vi "Actor Core.vi"(8 "error in":errorcluster, 11 "Off-Grid in":refnum<class "Off-Grid.lvclass">) -> (0 "error out":errorcluster, 3 "Actor out":refnum<class "Actor.lvclass">)   [LabVIEW 2018, in "Off-Grid Actor.lvlib" / "Off-Grid.lvclass"]
doc: "(<B>Filename</B>: Actor Framework.lvlib:Actor.lvclass:Actor Core.vi)\n\nReceives messages to the actor, reacts to them, and initiates any error handling that may shut the actor down.\n\nDescendant classes may override this VI to append parallel tasks for the actor to complete while it handles messages. Overrides use the Call Parent Method node."
uses:
  Off-Grid.lvclass
  C:/Users/Administrator/Desktop/LabVIEW EMS/Optimization/Generic Optimization Actor/Generic Optimization/Generic Optimization.lvclass
  C:/Program Files (x86)/National Instruments/LabVIEW 2018/vi.lib/ActorFramework/Actor/Actor.lvclass
  C:/Users/Administrator/Desktop/LabVIEW EMS/EMS Generic Actor/EMS Generic/EMS Generic.lvclass
  <vilib>/ActorFramework/Actor/Actor.lvclass
  Generic Optimization Actor/Generic Optimization Messages/Find and Rejoin Devices Msg/Find and Rejoin Devices Msg.lvclass
  C:/Program Files (x86)/National Instruments/LabVIEW 2018/vi.lib/ActorFramework/Message/Message.lvclass
  <vilib>/ActorFramework/Actor/Actor.lvclass/Actor.ctl
  <vilib>/ActorFramework/Message Enqueuer/Message Enqueuer.lvclass/Message Enqueuer.ctl
  EMS Generic Actor/EMS Generic/EMS Generic.lvclass/EMS Generic.ctl
  Generic Optimization Actor/Generic Optimization/Optimization Controls/PCC Data.ctl
  <vilib>/ActorFramework/Message Enqueuer/Init from Existing Queue.vi
  <vilib>/ActorFramework/Message Enqueuer/Message Enqueuer.lvclass
  Generic Optimization Actor/Generic Optimization/Generic Optimization.lvclass
  EMS Generic Actor/EMS Generic/EMS Generic.lvclass
panel:
  out "Solution Result":string="Waiting"
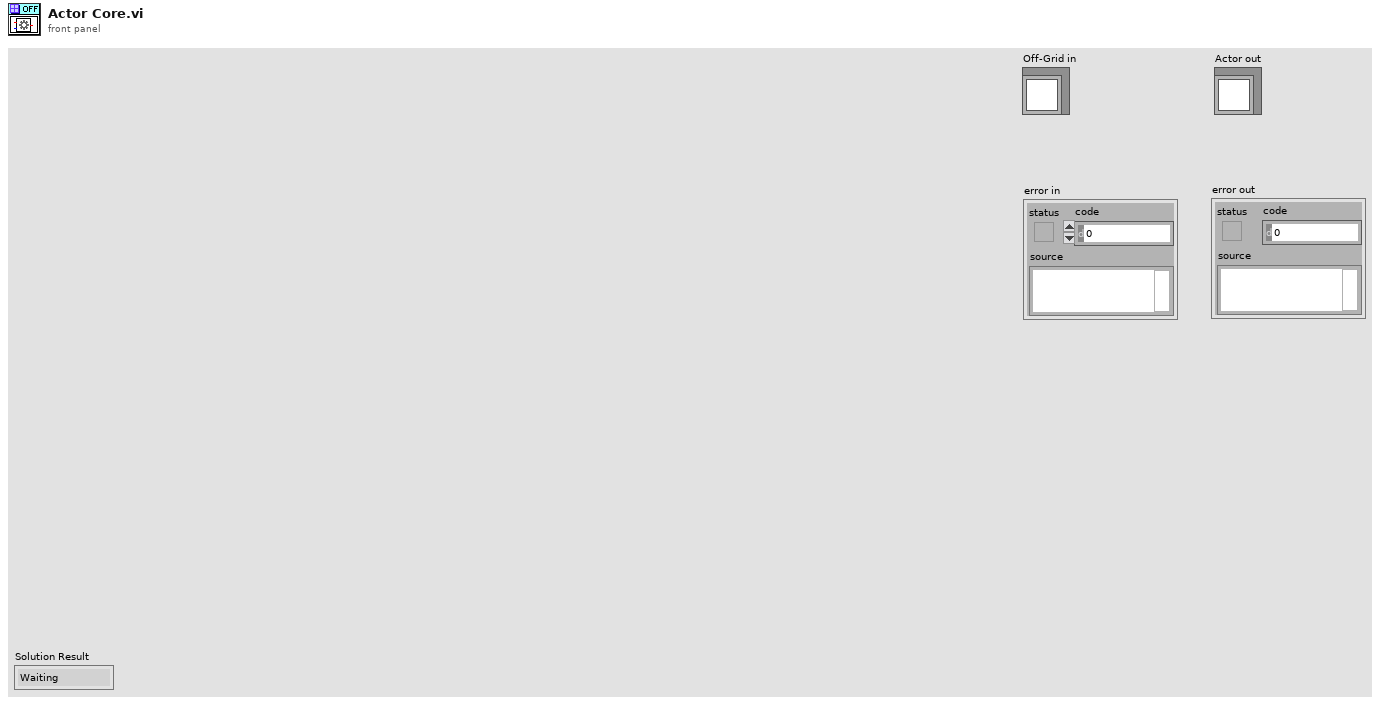
[diagram p1: front panel]
types:
  T1 = typedef "CSEISMIC DDS.lvlib/CSEISMIC DDS.lvclass/DeviceID.ctl" = string
  T2 = typedef "Generic Optimization Actor.lvlib/Generic Optimization.lvclass/Bus by ID.ctl" = cluster{"DeviceID":T1, "Bus ID":dbl}
  T3 = typedef "Generic Optimization Actor.lvlib/Generic Optimization.lvclass/Electrical Network Optimization Data.ctl" = cluster{"From_Bus":dbl, "To_Bus":dbl, "Network Resistance":dbl, "Network Reactance":dbl, "Power Flow Limits":dbl[], "Linear Piecewise Power Flow":dbl[], "Reactive Flow Limit":dbl[], "Linear Piecewise Reactive Flow":dbl[]}
  T4 = typedef "Generic Optimization Actor.lvlib/Generic Optimization.lvclass/PCC Data.ctl" = cluster{"PCC_max":dbl[], "PCC_min":dbl[], "QCC_max":dbl[], "QCC_min":dbl[]}
  T5 = typedef "EMS Generic Actor.lvlib/EMS Generic.lvclass/Global Configuration.ctl" = cluster{"Microgrid ID":u8, "VF Device ID":T1, "Ongrid VF Priority":T1[], "Offgrid VF Priority":T1[], "AutoSwap Offgrid VF":u32, "AutoSwap Offgrid VF Delay (sec)":dbl, "AutoSwap Resynch VF":u32, "PCC Device ID":T1, "Device ID Array":T1[], "Nominal Voltage":dbl, "Nominal Frequency":dbl, "Resynch Timeout (sec)":dbl, "Island VF Activate Timeout (sec)":dbl, "Island PCC Target Power (kW)":dbl, "Island PCC Target Power Timeout (sec)":dbl, "Island Grid Settle Time (sec)":dbl, "Island PCC Failure Timeout (sec)":dbl, "Activation Devices Present Timeout (sec)":dbl, "Activation Devices Activated Timeout (sec)":dbl, "Blackstart VF GenMode Wait (sec)":dbl, "Blackstart VF DERCtrl Wait (sec)":dbl, "Blackstart Success Wait (sec)":dbl, "OnGrid Optimization Delay (sec)":dbl, "OffGrid Optimization Delay (sec)":dbl, "Resynch Frequency (Hz)":dbl, "Optimization Path":string}
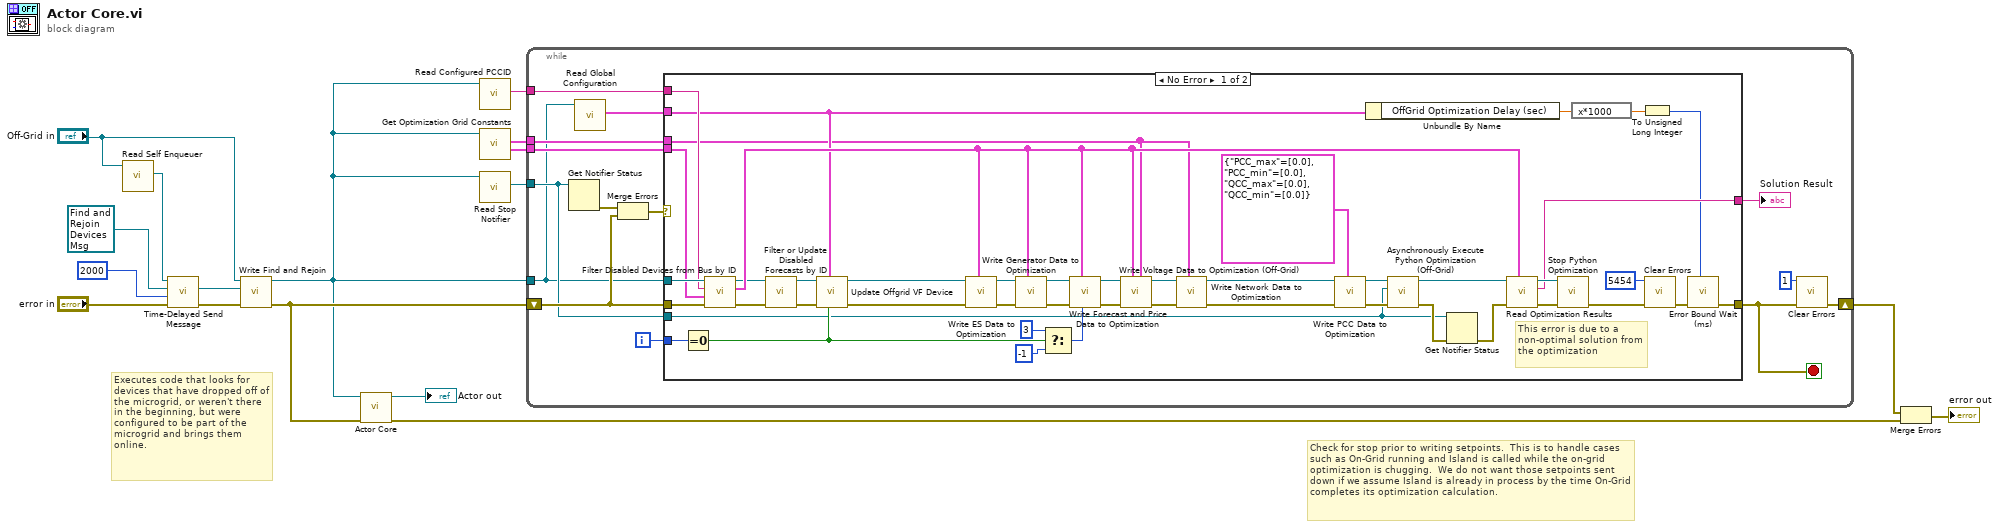
[diagram p0: block diagram]
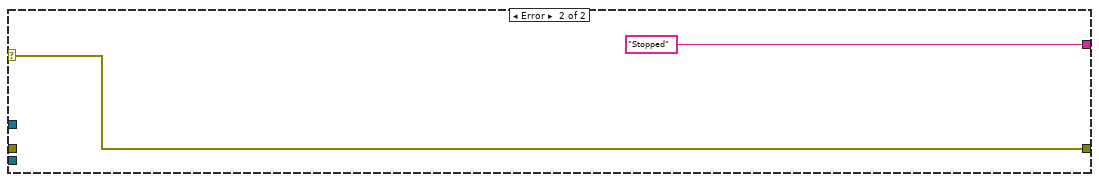
[diagram p2: hidden frame]
diagram:
  # "Executes code that looks for devices that have dropped off of the microgrid, or weren't there in the beginning, but were configured to be part of the microgrid and brings them online."
  # "Check for stop prior to writing setpoints.  This is to handle cases such as On-Grid running and Island is called while the on-grid optimization is chugging.  We do not want those setpoints sent down if we assume Island is already in process by the time On-Grid completes its optimization calculation."
  n1 = call <vilib>:"Read Self Enqueuer.vi"("Actor"="Off-Grid in") -> ("Self Enqueuer"=w8:refnum<class "Message Enqueuer.lvclass">)  [unwired: 10 in]
  n2 = call <vilib>:"Time-Delayed Send Message.vi"("error in (no error)"="error in", "Milliseconds To Wait"=2000, "Message"=refnum<class "Find and Rejoin Devices Msg.lvclass"> refnum ("Generic Optimization Actor.lvlib:Find and Rejoin Devices Msg.lvclass"), "Message Enqueuer"=w8) -> ("error out"=w5:errorcluster, "Delivery Notifier"=w3:refnum<notifier>)  [unwired: 6 in]
  n3 = call "Write Find and Rejoin.vi"("error in"=w5, "Find and Rejoin"=w3, "Generic Optimization in"="Off-Grid in") -> ("error out"=w4:errorcluster, "Generic Optimization out"=w1:refnum<class "Off-Grid.lvclass">)  [unwired: 7 in]
  n4 = call-parent "Actor Core.vi"("error in"=w4, "Actor in"=w1) -> ("error out"=w12:errorcluster, "Actor out"=→"Actor out":refnum<class "Actor.lvclass">)  [unwired: 8 in]
  n5 = call "Read Configured PCCID.vi"("EMS Generic in"=w1) -> ("PCCID"=w10:T1)  [unwired: 8 in, 2 out]
  n6 = call "Get Optimization Grid Constants.vi"("Generic Optimization in"=w1) -> ("Bus by ID"=w14:T2[], "Network Data"=w13:T3[])  [unwired: 8 in, 1 out]
  n7 = call "Read Stop Notifier.vi"("EMS Generic in"=w1) -> ("stop"=w16:refnum<notifier>)  [unwired: 9 in, 1 out]
  n8 = while {
    tunnel: w14 -> [w30]
    tunnel: w13 -> [w31]
    tunnel: w1 -> [w19]
    tunnel: w16 -> [w25]
    shift-right: [w22] -> w15
    shift-left: w4 -> [w27]
    tunnel: w10 -> [w21]
    i -> [w20]
    stop <- w23 stop-if-true
    n9 = Get Notifier Status(notifier=w25) -> (error out=w28:errorcluster)  [unwired: 1 in, 4 out]
    n10 = call "Read Global Configuration.vi"("EMS Generic in"=w19) -> ("Global Configuration"=w18:T5)  [unwired: 8 in, 2 out]
    n11 = Merge Errors(w28, w27) -> (w26:errorcluster)
    n12 = case shown="No Error" w26 {
      selector: w26 -> [_ w77]
      tunnel: w31 -> [w32 _]
      tunnel: w19 -> [w54 _]
      tunnel: w27 -> [w53 _]
      tunnel: w30 -> [w51 _]
      tunnel: [w43 w77] -> w23
      tunnel: [w61 "Stopped" ("Solution Result")] -> w29
      tunnel: w25 -> [w33 _]
      tunnel: w21 -> [w52 _]
      tunnel: w20 -> [w47 _]
      tunnel: w18 -> [w35 _]
      frame No Error {
        # "This error is due to a non-optimal solution from the optimization"
        n13 = Equal To 0?(x=w47) -> (x = 0?=w34:bool)
        n14 = call "Filter Disabled Devices from Bus by ID.vi"("error in"=w53, "BusData"=w51, "PCCID"=w52, "Generic Optimization in"=w54) -> ("dup error out"=w49:errorcluster, "Filtered Bus by ID"=w50:T2[], "Generic Optimization out"=w48:refnum<class "Off-Grid.lvclass">)  [unwired: 5 in]
        n15 = call "Filter or Update Disabled Forecasts by ID.vi"("error in"=w49, "Generic Optimization in"=w48) -> ("dup error out"=w39:errorcluster, "Generic Optimization out"=w37:refnum<class "Off-Grid.lvclass">)  [unwired: 8 in]
        n16 = call "Update Offgrid VF Device.vi"("Reset Swap Delay"=w34, "Global Configuration"=w35, "error in"=w39, "Off-Grid in"=w37) -> ("error out"=w38:errorcluster, "Off-Grid out"=w36:refnum<class "Off-Grid.lvclass">)  [unwired: 6 in]
        n17 = call "Write ES Data to Optimization.vi"("Bus by ID"=w50, "error in"=w38, "Generic Optimization in"=w36) -> ("error out"=w73:errorcluster, "Generic Optimization out"=w72:refnum<class "Off-Grid.lvclass">)  [unwired: 7 in]
        n18 = call "Write Generator Data to Optimization.vi"("Bus by ID"=w50, "error in"=w73, "Generic Optimization in"=w72) -> ("error out"=w76:errorcluster, "Generic Optimization out"=w71:refnum<class "Off-Grid.lvclass">)  [unwired: 7 in]
        n19 = Select(t=3, s=w34, f=-1 ("Max Forecast Length (-1: no limit)")) -> (s? t:f=w44:i32)
        n20 = call "Write Forecast and Price Data to Optimization.vi"("Max Forecast Length (-1: no limit)"=w44, "Bus by ID"=w50, "error in"=w76, "Generic Optimization in"=w71) -> ("error out"=w75:errorcluster, "Generic Optimization out"=w70:refnum<class "Off-Grid.lvclass">)  [unwired: 6 in]
        n21 = call "Write Voltage Data to Optimization (Off-Grid).vi"("Network Data Array"=w32, "Bus by ID"=w50, "error in"=w75, "Off-Grid Optimization in"=w70) -> ("error out"=w74:errorcluster, "Off-Grid Optimization out"=w69:refnum<class "Off-Grid.lvclass">)  [unwired: 6 in]
        n22 = call "Write Network Data to Optimization.vi"("Network Data Array"=w32, "error in"=w74, "Generic Optimization in"=w69) -> ("error out"=w60:errorcluster, "Generic Optimization out"=w58:refnum<class "Off-Grid.lvclass">)  [unwired: 7 in]
        n23 = call "Write PCC Data to Optimization.vi"("PCC Data"=T4 {"PCC_max"=[0.0], "PCC_min"=[0.0], "QCC_max"=[0.0], "QCC_min"=[0.0]}, "error in"=w60, "Generic Optimization in"=w58) -> ("error out"=w59:errorcluster, "Generic Optimization out"=w57:refnum<class "Off-Grid.lvclass">)  [unwired: 7 in]
        n24 = Unbundle By Name(w35) -> ("OffGrid Optimization Delay (sec)"=w42:dbl)
        n25 = call "Asynchronously Execute Python Optimization (Off-Grid).vi"("error in"=w59, "Stop Notifier"=w33, "Off-Grid in"=w57) -> ("error out"=w63:errorcluster, "Off-Grid out"=w68:refnum<class "Off-Grid.lvclass">)  [unwired: 7 in]
        n26 = Get Notifier Status(notifier=w33, error in (no error)=w63) -> (error out=w62:errorcluster)  [unwired: 4 out]
        n27 = call "Read Optimization Results.vi"("Bus by ID Array"=w50, "error in"=w62, "Generic Optimization in"=w68) -> ("error out"=w66:errorcluster, "Solution Result"=w61:string, "Generic Optimization out"=w67:refnum<class "Off-Grid.lvclass">)  [unwired: 6 in]
        n28 = call "Stop Python Optimization.vi"("error in"=w66, "Generic Optimization in"=w67) -> ("error out"=w56:errorcluster)  [unwired: 8 in, 1 out]
        n29 = expression code="x*1000"(w42) -> (w41:dbl)
        n30 = To Unsigned Long Integer(number=w41) -> (unsigned 32bit integer=w40:u32)
        n31 = call <vilib>:"Clear Errors.vi"("error in (no error)"=w56, "specific error code to clear (0: all)"=5454) -> ("error out"=w65:errorcluster)  [unwired: 4 in, 1 out]
        n32 = call "Error Bound Wait (ms).vi"("milliseconds to wait (100)"=w40, "error in"=w65) -> ("error out"=w43:errorcluster)  [unwired: 9 in]
      }
      frame Error {
      }
    }
    "Solution Result" <- w29
    n33 = call <vilib>:"Clear Errors.vi"("error in (no error)"=w23, "specific error code to clear (0: all)"=1) -> ("error out"=w22:errorcluster)  [unwired: 4 in, 1 out]
  }
  n34 = Merge Errors(w15, w12) -> (→"error out":errorcluster)
